vi "Stop.vi"(2 "Close FP":bool) -> (0 "Stop Now?":bool)   [LabVIEW 2022 SP3]
panel:
  in  "Stop Now?":bool
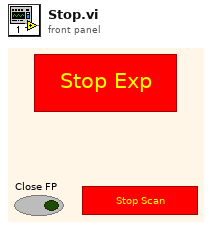
[diagram p1: front panel]
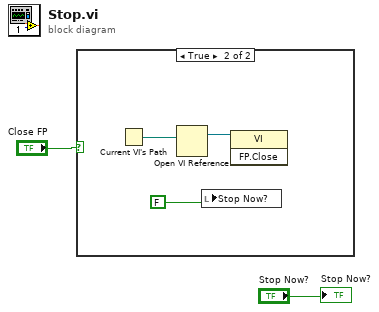
[diagram p0: block diagram]
diagram:
  n1 = case shown="True" "Close FP" {
    frame False {
    }
    frame True {
      n2 = Current VI's Path() -> (path=w5:path)
      n3 = Open VI Reference(vi path=w5) -> (vi reference=w4:refnum<vi>)  [unwired: 2 in, 4 out]
      n4 = local write "Stop Now?"(FALSE) -> ()
      n5 = invoke class="VI" method="FP.Close"(reference=w4) -> ()  [unwired: 2 in, 3 out]
    }
  }
  "Stop Now?" <- "Stop Now?"
